vi "get_project.vi"(11 "path":string) -> (0 "error out":errorcluster, 3 "text":string)   [LabVIEW 2026, in "G-AI Core.lvlib"]
doc: "Returns the XML content of a LabVIEW Project- or Library-File specified by path. (lvlib, lvproj, lvclass filetypes). To get a full projects multiple calls may be necessary to get all nested libraries."
uses:
  G-AI Core.lvlib
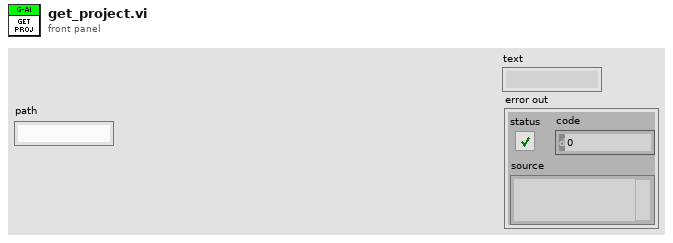
[diagram p1: front panel]
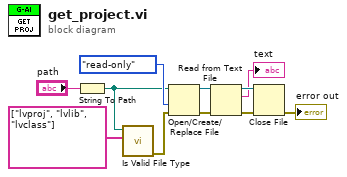
[diagram p0: block diagram]
diagram:
  n1 = String To Path(string="path") -> (path=w3:path)
  n2 = call "Is Valid File Type.vi"("y"=string[] ["lvproj", "lvlib", "lvclass"], "Path"=w3) -> ("error out"=w2:errorcluster)  [unwired: 9 in]
  n3 = Open/Create/Replace File(file path (use dialog)=w3, error in=w2, access (0:read/write)=enum16{"read/write", "read-only", "write-only"}."read-only") -> (refnum out=w10:refnum<file>, error out=w9:errorcluster)  [unwired: 3 in, 1 out]
  n4 = Read from Text File(file (use dialog)=w10, error in=w9) -> (refnum out=w8:refnum<file>, text=→"text":string, error out=w7:errorcluster)  [unwired: 2 in, 1 out]
  n5 = Close File(refnum=w8, error in=w7) -> (error out=→"error out":errorcluster)  [unwired: 1 out]
